vi "Framework_S_Para_Data_Types.vi"() -> ()   [LabVIEW 2020]
panel:
  out "S-parameters":cdb[][](array[numeric]) format="%#.6g"
  out "Z0 (Ohm)":cdb
  out "Frequencies (Hz)":dbl[](array[numeric])
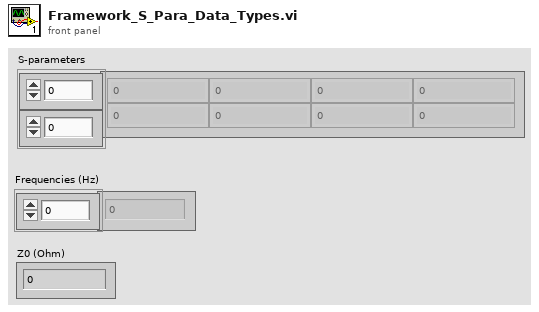
[diagram p1: front panel]
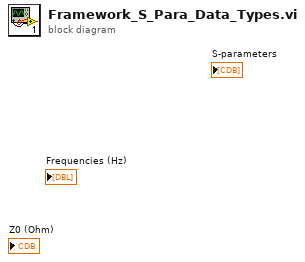
[diagram p0: block diagram]
diagram:
